vi "运维调试_五参数.vi"() -> ()   [LabVIEW 2016, in "斯坦道多参数.lvlib"]
uses:
  <vilib>/Utility/miscctls.llb/LVPointTypeDef.ctl
  <vilib>/Utility/config.llb/NI_LVConfig.lvlib
panel:
  out "运行状态":u16(ring) items=["空闲", "水样测试", "标样核查"]
  in  "叶绿素a校准":bool
  in  "停止":bool
  in  "标样核查":bool
  in  "水样测试":bool
  in  "open MB":bool
  in  "设置":bool
  in  "水温校准":bool
  in  "浊度校准":bool
  in  "溶解氧校准":bool
  in  "电导率校准":bool
  in  "pH校准":bool
  in  "探头校正返回":bool
  in  "探头校正":bool
  out "检测值":T1
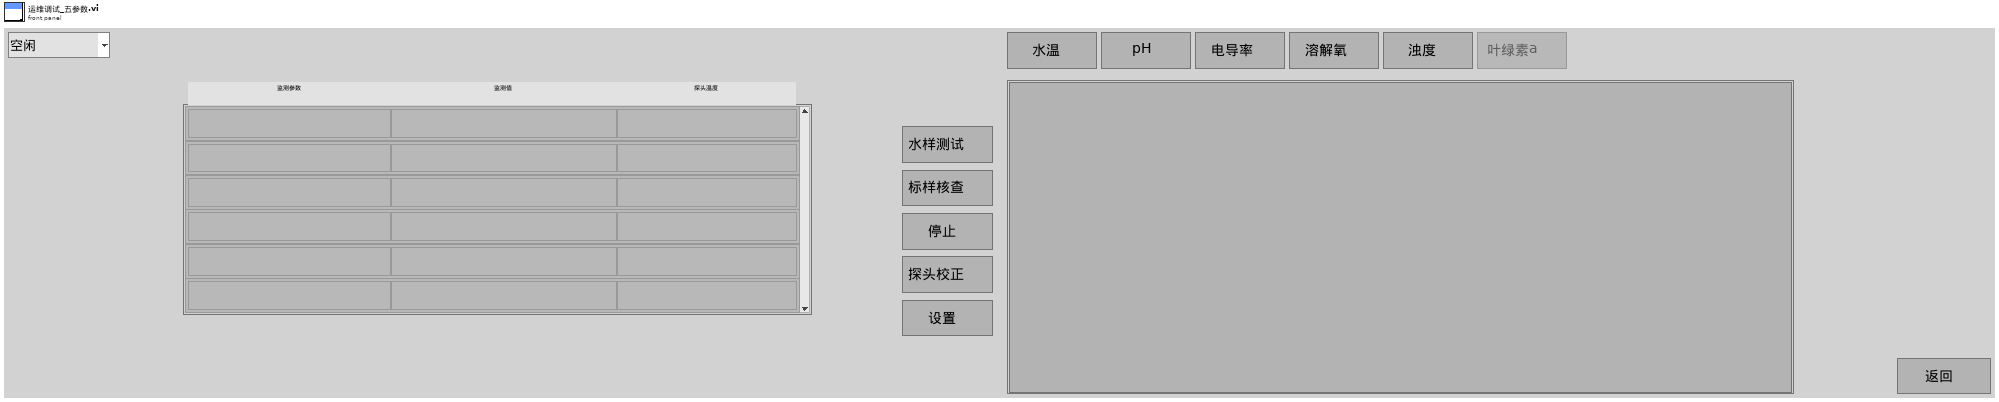
[diagram p1: front panel]
types:
  T1 = typedef "斯坦道多参数.lvlib/检测值.ctl" = cluster{"监测参数1":string, "浓度1":string, "探头温度1":string}[]
  T2 = typedef "LVPointTypeDef.ctl" = cluster{"Horizontal":i16, "Vertical":i16}
  T3 = cluster{"电极状态标志":u16, "电极型号标志":u16, "酸碱度测量值":sgl, "温度测量值":sgl, "酸碱度信号值":sgl, "温度信号值":sgl, "酸碱度偏移修正值":sgl, "温度偏移修正值":sgl, "手动温度补偿值":sgl, "酸碱度电极零点":sgl, "酸碱度电极斜率":sgl, "第1点标准值记录":sgl, "第1点信号值记录":sgl, "第1点温度值记录":sgl, "第2点标准值记录":sgl, "第2点信号值记录":sgl, "第2点温度值记录":sgl, "命令滤波设定":u16, "温度模式":enum16{"ATC", "MTC"}, "生产批次":u16, "电极序号":u16, "串口地址":u16, "串口波特率":enum16{"9600", "19200", "115200"}, "串口校验位":enum16{"NONE", "ODD", "EVEN"}, "串口停止位":enum16{"1bit", "2bit"}, "第一点标准值":sgl, "第二点标准值":sgl}
  T4 = cluster{"电极状态标志":u16, "电极型号标志":u16, "电导率测量值":sgl, "温度测量值":sgl, "电导率信号值":sgl, "温度信号值":sgl, "温度补偿系数":sgl, "电导率偏移修正值":sgl, "温度偏移修正值":sgl, "手动温度补偿值":sgl, "电导率电极零点":sgl, "电导率电极斜率":sgl, "命令滤波设定":u16, "温度模式":enum16{"ATC", "MTC"}, "生产批次":u16, "电极序号":u16, "串口地址":u16, "串口波特率":enum16{"9600", "19200", "115200"}, "串口校验位":enum16{"NONE", "ODD", "EVEN"}, "串口停止位":enum16{"1bit", "2bit"}, "第一点标准值":sgl, "第二点标准值":sgl}
  T5 = cluster{"监测参数1":string, "浓度1":string, "探头温度1":string}[]
  T6 = enum8{"Enabled", "Disabled", "Disabled and Grayed Out"}
  T7 = cluster{"CH":u16, "监测值":dbl, "监测信号值":dbl, "温度偏移修正值":sgl}
  T8 = typedef "NI_LVConfig.lvlib/Config Data RefNum.ctl" = refnum<k1>
  T9 = cluster{"baud rate (bps)":u32, "stop bits":u16, "parity":u16, "flow control":u16, "timeout":u32, "retries":i32}
  T10 = enum32{"Bad", "Idle", "Run top level", "Running"}
  T11 = cluster{"数据保存间隔":dbl, "水温标样值":dbl, "pH标样值":dbl, "溶解氧标样值":dbl, "电导率标样值":dbl, "浊度标样值":dbl}
  T12 = cluster{"Temp":bool, "pH":bool, "DO":bool, "Cond":bool, "Turb":bool, "叶绿素a启用":bool}
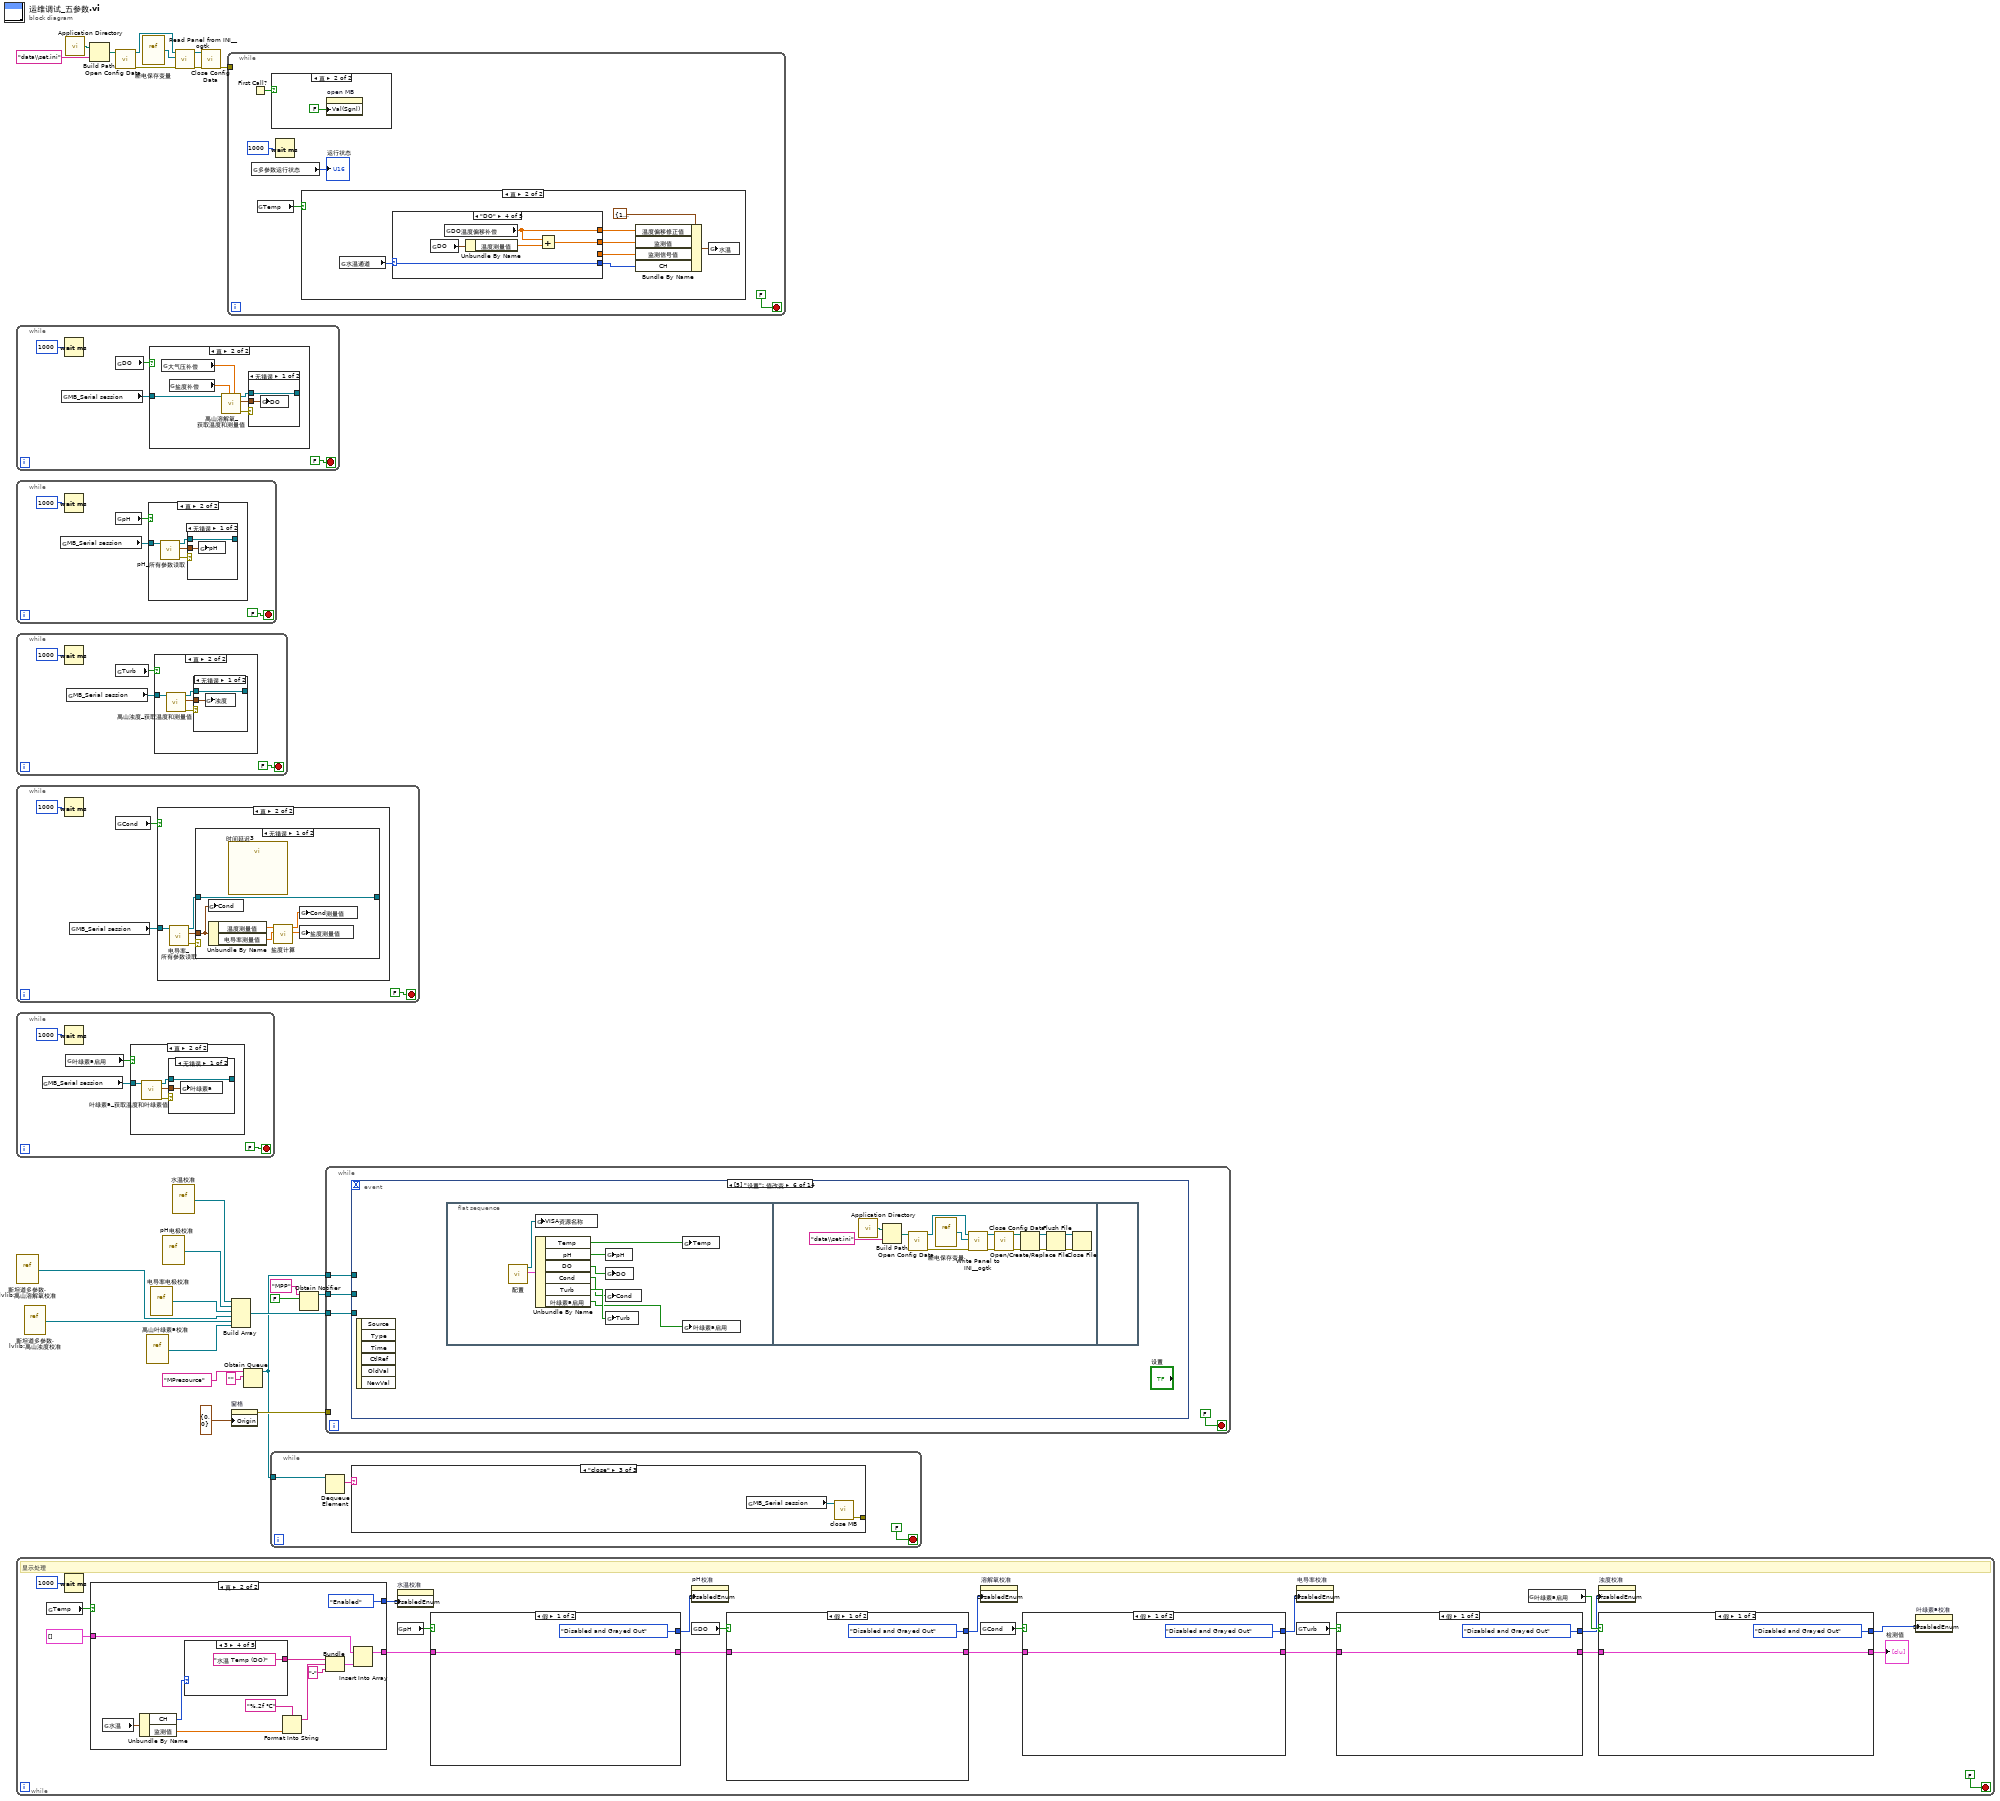
[diagram p0: block diagram]
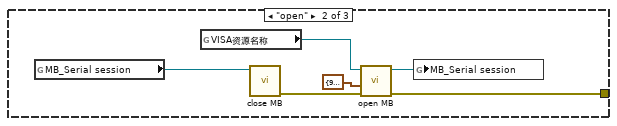
[diagram p3: hidden frame]
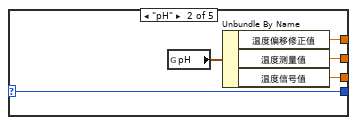
[diagram p16: hidden frame]
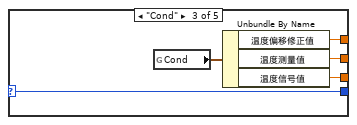
[diagram p17: hidden frame]
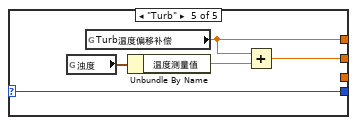
[diagram p18: hidden frame]
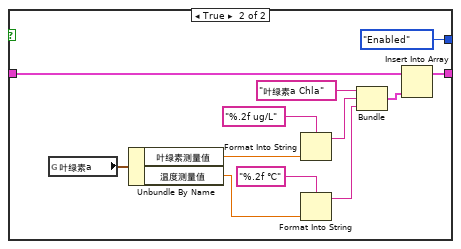
[diagram p20: hidden frame]
diagram:
  n1 = while {
    stop <- FALSE stop-if-true
    n2 = global read "多参数全局变量.vi" "MB_Serial session"() -> (w25:refnum<class "MB_Master_Serial.lvclass">)
    n3 = Wait (ms)(milliseconds to wait=u32 1000 ("等待时间（毫秒）")) -> ()  [unwired: 1 out]
    n4 = global read "断电保存变量.vi" "DO"() -> (w26:bool)
    n5 = case shown="真" w26 {
      tunnel: w25 -> [_ w31]
      frame False {
      }
      frame True {
        n6 = global read "断电保存变量.vi" "大气压补偿"() -> (w30:dbl)
        n7 = global read "断电保存变量.vi" "盐度补偿"() -> (w29:dbl)
        n8 = call "禹山溶解氧_获取温度和测量值.vi"("大气压补偿"=w30, "盐度补偿"=w29, "MB_Serial session in"=w31) -> ("error out"=w33:errorcluster, "输出值"=w34:cluster{"温度测量值":sgl, "DO%":sgl, "DOmg/L":sgl}, "MB_Serial session out"=w32:refnum<class "MB_Master_Serial.lvclass">)  [unwired: 6 in]
        n9 = case shown="无错误" w33 {
          tunnel: w34 -> [w35 _]
          tunnel: w32 -> [w36 w37]
          tunnel: [w36 w37] -> _
          frame No Error {
            n10 = global write "禹山过程全局变量.vi" "DO"(w35) -> ()
          }
          frame Error {
          }
        }
      }
    }
  }
  n11 = while {
    stop <- FALSE stop-if-true
    n12 = global read "多参数全局变量.vi" "MB_Serial session"() -> (w38:refnum<class "MB_Master_Serial.lvclass">)
    n13 = Wait (ms)(milliseconds to wait=u32 1000 ("等待时间（毫秒）")) -> ()  [unwired: 1 out]
    n14 = global read "断电保存变量.vi" "pH"() -> (w40:bool)
    n15 = case shown="真" w40 {
      tunnel: w38 -> [_ w42]
      frame False {
      }
      frame True {
        n16 = call "pH_所有参数读取.vi"("MB_Serial session in"=w42) -> ("error out"=w44:errorcluster, "输出值"=w45:T3, "MB_Serial session out"=w43:refnum<class "MB_Master_Serial.lvclass">)  [unwired: 8 in]
        n17 = case shown="无错误" w44 {
          tunnel: w45 -> [w47 _]
          tunnel: w43 -> [w46 w48]
          tunnel: [w46 w48] -> _
          frame No Error {
            n18 = global write "国弘过程全局变量.vi" "pH"(w47) -> ()
          }
          frame Error {
          }
        }
      }
    }
  }
  n19 = while {
    stop <- FALSE stop-if-true
    n20 = Wait (ms)(milliseconds to wait=u32 1000 ("等待时间（毫秒）")) -> ()  [unwired: 1 out]
    n21 = global read "多参数全局变量.vi" "MB_Serial session"() -> (w49:refnum<class "MB_Master_Serial.lvclass">)
    n22 = global read "断电保存变量.vi" "Turb"() -> (w51:bool)
    n23 = case shown="真" w51 {
      tunnel: w49 -> [_ w53]
      frame False {
      }
      frame True {
        n24 = call "禹山浊度_获取温度和测量值.vi"("MB_Serial session in"=w53) -> ("error out"=w55:errorcluster, "输出值"=w56:cluster{"温度测量值":sgl, "浊度":sgl}, "MB_Serial session out"=w54:refnum<class "MB_Master_Serial.lvclass">)  [unwired: 8 in]
        n25 = case shown="无错误" w55 {
          tunnel: w56 -> [w57 _]
          tunnel: w54 -> [w58 w59]
          tunnel: [w58 w59] -> _
          frame No Error {
            n26 = global write "禹山过程全局变量.vi" "浊度"(w57) -> ()
          }
          frame Error {
          }
        }
      }
    }
  }
  n27 = while {
    stop <- FALSE stop-if-true
    n28 = Wait (ms)(milliseconds to wait=u32 1000 ("等待时间（毫秒）")) -> ()  [unwired: 1 out]
    n29 = global read "多参数全局变量.vi" "MB_Serial session"() -> (w60:refnum<class "MB_Master_Serial.lvclass">)
    n30 = global read "断电保存变量.vi" "Cond"() -> (w62:bool)
    n31 = case shown="真" w62 {
      tunnel: w60 -> [_ w64]
      frame False {
      }
      frame True {
        n32 = call "电导率_所有参数读取.vi"("MB_Serial session in"=w64) -> ("error out"=w66:errorcluster, "输出值"=w67:T4, "MB_Serial session out"=w65:refnum<class "MB_Master_Serial.lvclass">)  [unwired: 8 in]
        n33 = case shown="无错误" w66 {
          tunnel: w67 -> [w72 _]
          tunnel: [w73 w74] -> _
          tunnel: w65 -> [w73 w74]
          frame No Error {
            n34 = global write "国弘过程全局变量.vi" "Cond"(w72) -> ()
            n35 = Unbundle By Name(w72) -> ("温度测量值"=w70:sgl, "电导率测量值"=w71:sgl)
            n36 = call "时间延迟3"() -> ()  [unwired: 11 in, 1 out]
            n37 = call "盐度计算.vi"("spCond"=w71, "Temp"=w70) -> ("saltresult"=w68:dbl, "cond"=w69:dbl)  [unwired: 8 in]
            n38 = global write "国弘过程全局变量.vi" "Cond测量值"(w69) -> ()
            n39 = global write "国弘过程全局变量.vi" "盐度测量值"(w68) -> ()
          }
          frame Error {
          }
        }
      }
    }
  }
  n40 = while {
    stop <- FALSE stop-if-true
    n41 = global read "多参数全局变量.vi" "MB_Serial session"() -> (w75:refnum<class "MB_Master_Serial.lvclass">)
    n42 = Wait (ms)(milliseconds to wait=u32 1000 ("等待时间（毫秒）")) -> ()  [unwired: 1 out]
    n43 = global read "断电保存变量.vi" "叶绿素a启用"() -> (w77:bool)
    n44 = case shown="真" w77 {
      tunnel: w75 -> [_ w79]
      frame False {
      }
      frame True {
        n45 = call "叶绿素a_获取温度和叶绿素值.vi"("MB_Serial session in"=w79) -> ("error out"=w81:errorcluster, "输出值"=w82:cluster{"温度测量值":sgl, "叶绿素测量值":sgl, "错误标志":u16}, "MB_Serial session out"=w80:refnum<class "MB_Master_Serial.lvclass">)  [unwired: 8 in]
        n46 = case shown="无错误" w81 {
          tunnel: w82 -> [w83 _]
          tunnel: w80 -> [w84 w85]
          tunnel: [w84 w85] -> _
          frame No Error {
            n47 = global write "禹山过程全局变量.vi" "叶绿素a"(w83) -> ()
          }
          frame Error {
          }
        }
      }
    }
  }
  n48 = vi-ref "斯坦道多参数.lvlib:禹山溶解氧校准.vi"() -> (w18:refnum<vi>)
  n49 = while {
    stop <- FALSE stop-if-true
    # "显示处理"
    n50 = global read "断电保存变量.vi" "Temp"() -> (w104:bool)
    n51 = Wait (ms)(milliseconds to wait=u32 1000 ("等待时间（毫秒）")) -> ()  [unwired: 1 out]
    n52 = case shown="真" w104 {
      tunnel: [w182 w184] -> w101
      tunnel: T5 [] ("数组") -> [w182 w185]
      tunnel: [T6."Disabled and Grayed Out" ("禁用") T6."Enabled" ("禁用")] -> w86
      frame False {
      }
      frame True {
        n53 = global read "国弘过程全局变量.vi" "水温"() -> (w193:T7)
        n54 = Unbundle By Name(w193) -> ("CH"=w190:u16, "监测值"=w191:dbl)
        n55 = case shown="3" w190 {
          tunnel: ["水温 Temp" ("监测参数1") "水温 Temp (pH)" ("监测参数1") "水温 Temp (Cond)" ("监测参数1") "水温 Temp (DO)" ("监测参数1") "水温 Temp (Turb)" ("监测参数1")] -> w189
          frame 0, Default {
          }
          frame 1 {
          }
          frame 2 {
          }
          frame 3 {
          }
          frame 4 {
          }
        }
        n56 = Format Into String(format string="%.2f ℃" ("格式字符串"), w191) -> (resulting string=w188:string)  [unwired: 2 in, 1 out]
        n57 = Bundle("监测参数1"=w189, w188, "探头温度1"="-") -> (w186:cluster{"监测参数1":string, string, "探头温度1":string})  [unwired: 1 in]
        n58 = Insert Into Array(array=w185, new element=w186) -> (w184:T5)  [unwired: 1 in]
      }
    }
    n59 = property on="水温校准" class="Bool"("DisabledEnum"=w86) -> ()  [unwired: 2 in, 2 out]
    n60 = global read "断电保存变量.vi" "pH"() -> (w102:bool)
    n61 = case shown="假" w102 {
      tunnel: [w168 w170] -> w99
      tunnel: w101 -> [w168 w172]
      tunnel: [T6."Disabled and Grayed Out" ("禁用") T6."Enabled" ("禁用")] -> w91
      frame False {
      }
      frame True {
        n62 = global read "国弘过程全局变量.vi" "pH"() -> (w180:T3)
        n63 = Unbundle By Name(w180) -> ("酸碱度测量值"=w179:sgl, "温度测量值"=w177:sgl)
        n64 = Format Into String(format string="%.2f" ("格式字符串"), w179) -> (resulting string=w173:string)  [unwired: 2 in, 1 out]
        n65 = Format Into String(format string="%.2f ℃" ("格式字符串"), w177) -> (resulting string=w175:string)  [unwired: 2 in, 1 out]
        n66 = Bundle("监测参数2"="酸碱度 pH", w173, w175) -> (w171:cluster{"监测参数2":string, string, string})  [unwired: 1 in]
        n67 = Insert Into Array(array=w172, new element=w171) -> (w170:T5)  [unwired: 1 in]
      }
    }
    n68 = property on="pH校准" class="Bool"("DisabledEnum"=w91) -> ()  [unwired: 2 in, 2 out]
    n69 = global read "断电保存变量.vi" "DO"() -> (w100:bool)
    n70 = case shown="假" w100 {
      tunnel: [w150 w153] -> w96
      tunnel: w99 -> [w150 w154]
      tunnel: [T6."Disabled and Grayed Out" ("禁用") T6."Enabled" ("禁用")] -> w90
      frame False {
      }
      frame True {
        n71 = global read "禹山过程全局变量.vi" "DO"() -> (w152:cluster{"温度测量值":sgl, "DO%":sgl, "DOmg/L":sgl})
        n72 = Unbundle By Name(w152) -> ("DOmg/L"=w163:sgl, "DO%"=w161:sgl, "温度测量值"=w165:sgl)
        n73 = Format Into String(format string="%.2f mg/L" ("格式字符串"), w163) -> (resulting string=w160:string)  [unwired: 2 in, 1 out]
        n74 = Format Into String(format string="(%.2f %%)" ("格式字符串"), w161) -> (resulting string=w159:string)  [unwired: 2 in, 1 out]
        n75 = Concatenate Strings(w160, w159) -> (w158:string)
        n76 = Format Into String(format string="%.2f ℃" ("格式字符串"), w165) -> (resulting string=w156:string)  [unwired: 2 in, 1 out]
        n77 = Bundle("监测参数2"="溶解氧 DO", w158, w156) -> (w155:cluster{"监测参数2":string, string, string})  [unwired: 1 in]
        n78 = Insert Into Array(array=w154, new element=w155) -> (w153:T5)  [unwired: 1 in]
      }
    }
    n79 = property on="溶解氧校准" class="Bool"("DisabledEnum"=w90) -> ()  [unwired: 2 in, 2 out]
    n80 = global read "断电保存变量.vi" "Cond"() -> (w98:bool)
    n81 = case shown="假" w98 {
      tunnel: w96 -> [w136 w140]
      tunnel: [w136 w138] -> w95
      tunnel: [T6."Disabled and Grayed Out" ("禁用") T6."Enabled" ("禁用")] -> w89
      frame False {
      }
      frame True {
        n82 = global read "国弘过程全局变量.vi" "Cond"() -> (w148:T4)
        n83 = Unbundle By Name(w148) -> ("电导率测量值"=w147:sgl, "温度测量值"=w145:sgl)
        n84 = Format Into String(format string="%.2f uS/cm" ("格式字符串"), w147) -> (resulting string=w141:string)  [unwired: 2 in, 1 out]
        n85 = Format Into String(format string="%.2f ℃" ("格式字符串"), w145) -> (resulting string=w142:string)  [unwired: 2 in, 1 out]
        n86 = Bundle("监测参数2"="电导率 Cond", w141, w142) -> (w139:cluster{"监测参数2":string, string, string})  [unwired: 1 in]
        n87 = Insert Into Array(array=w140, new element=w139) -> (w138:T5)  [unwired: 1 in]
      }
    }
    n88 = property on="电导率校准" class="Bool"("DisabledEnum"=w89) -> ()  [unwired: 2 in, 2 out]
    n89 = global read "断电保存变量.vi" "Turb"() -> (w97:bool)
    n90 = case shown="假" w97 {
      tunnel: w95 -> [w122 w127]
      tunnel: [w122 w125] -> w94
      tunnel: [T6."Disabled and Grayed Out" ("禁用") T6."Enabled" ("禁用")] -> w88
      frame False {
      }
      frame True {
        n91 = global read "禹山过程全局变量.vi" "浊度"() -> (w124:cluster{"温度测量值":sgl, "浊度测量值":sgl})
        n92 = Unbundle By Name(w124) -> ("浊度测量值"=w131:sgl, "温度测量值"=w133:sgl)
        n93 = Format Into String(format string="%.2f NTU" ("格式字符串"), w131) -> (resulting string=w129:string)  [unwired: 2 in, 1 out]
        n94 = Format Into String(format string="%.2f ℃" ("格式字符串"), w133) -> (resulting string=w130:string)  [unwired: 2 in, 1 out]
        n95 = Bundle("监测参数2"="浊度 Turb", w129, w130) -> (w126:cluster{"监测参数2":string, string, string})  [unwired: 1 in]
        n96 = Insert Into Array(array=w127, new element=w126) -> (w125:T5)  [unwired: 1 in]
      }
    }
    n97 = global read "断电保存变量.vi" "叶绿素a启用"() -> (w92:bool)
    n98 = property on="浊度校准" class="Bool"("DisabledEnum"=w88) -> ()  [unwired: 2 in, 2 out]
    n99 = case shown="假" w92 {
      tunnel: w94 -> [w108 w115]
      tunnel: [w108 w113] -> w93
      tunnel: [T6."Disabled and Grayed Out" ("禁用") T6."Enabled" ("禁用")] -> w87
      frame False {
      }
      frame True {
        n100 = global read "禹山过程全局变量.vi" "叶绿素a"() -> (w112:cluster{"温度测量值":sgl, "叶绿素测量值":sgl, "错误标志":u16})
        n101 = Unbundle By Name(w112) -> ("叶绿素测量值"=w111:sgl, "温度测量值"=w110:sgl)
        n102 = Format Into String(format string="%.2f ug/L" ("格式字符串"), w111) -> (resulting string=w117:string)  [unwired: 2 in, 1 out]
        n103 = Format Into String(format string="%.2f ℃" ("格式字符串"), w110) -> (resulting string=w118:string)  [unwired: 2 in, 1 out]
        n104 = Bundle("监测参数2"="叶绿素a Chla", w117, w118) -> (w114:cluster{"监测参数2":string, string, string})  [unwired: 1 in]
        n105 = Insert Into Array(array=w115, new element=w114) -> (w113:T5)  [unwired: 1 in]
      }
    }
    "检测值" <- w93
    n106 = property on="叶绿素a校准" class="Bool"("DisabledEnum"=w87) -> ()  [unwired: 2 in, 2 out]
  }
  n107 = vi-ref "斯坦道多参数.lvlib:禹山浊度校准.vi"() -> (w17:refnum<vi>)
  n108 = call <vilib>:"Application Directory.vi"() -> ("Application Directory"=w12:path)
  n109 = Build Path(base path=w12, name or relative path="data\\set.ini" ("名称或相对路径")) -> (appended path=w11:path)
  n110 = call <vilib>:"Open Config Data.vi"("configuration file path"=w11) -> ("error out"=w15:errorcluster, "refnum"=w16:T8)  [unwired: 8 in, 1 out]
  n111 = vi-ref "断电保存变量.vi"() -> (w9:refnum<vi>)
  n112 = vi-ref "禹山叶绿素a校准.vi"() -> (w7:refnum<vi>)
  n113 = vi-ref "电导率电极校准.vi"() -> (w19:refnum<vi>)
  n114 = vi-ref "pH电极校准.vi"() -> (w20:refnum<vi>)
  n115 = vi-ref "水温校准.vi"() -> (w21:refnum<vi>)
  n116 = call <userlib>:"Read Panel from INI__ogtk.vi"("error in (no error)"=w15, "VI ref"=w9, "refnum"=w16) -> ("error out"=w13:errorcluster, "refnum out"=w14:T8)  [unwired: 7 in]
  n117 = call <vilib>:"Close Config Data.vi"("error in (no error)"=w13, "refnum"=w14) -> ("error out"=w8:errorcluster)  [unwired: 8 in, 1 out]
  n118 = while {
    tunnel: w8 -> [_]
    stop <- FALSE stop-if-true
    n119 = First Call?() -> (First Call?: T/F=w201:bool)
    n120 = global read "多参数全局变量.vi" "多参数运行状态"() -> (→"运行状态":u16)
    n121 = global read "断电保存变量.vi" "Temp"() -> (w200:bool)
    n122 = case shown="真" w201 {
      frame False {
      }
      frame True {
        n123 = property on="open MB" class="Bool (严格)"("Val(Sgnl)"=FALSE ("值(信号)")) -> ()  [unwired: 2 in, 2 out]
      }
    }
    n124 = Wait (ms)(milliseconds to wait=u32 1000 ("等待时间（毫秒）")) -> ()  [unwired: 1 out]
    n125 = case shown="真" w200 {
      frame False {
      }
      frame True {
        n126 = global read "断电保存变量.vi" "水温通道"() -> (w210:enum16{"NULL", "pH", "Cond", "DO", "Turb"})
        n127 = case shown="\"DO\"" w210 {
          selector: w210 -> [w211 w216 w221 w226 w231]
          tunnel: [w211 w216 w221 w226 w231] -> w209
          tunnel: [_ w214 w219 w222 w227] -> w208
          tunnel: [_ w213 w218 _ _] -> w207
          tunnel: [_ w212 w217 w223 w229] -> w204
          frame "NULL", Default {
          }
          frame "pH" {
            n128 = global read "国弘过程全局变量.vi" "pH"() -> (w215:T3)
            n129 = Unbundle By Name(w215) -> ("温度偏移修正值"=w212:sgl, "温度测量值"=w214:sgl, "温度信号值"=w213:sgl)
          }
          frame "Cond" {
            n130 = global read "国弘过程全局变量.vi" "Cond"() -> (w220:T4)
            n131 = Unbundle By Name(w220) -> ("温度偏移修正值"=w217:sgl, "温度测量值"=w219:sgl, "温度信号值"=w218:sgl)
          }
          frame "DO" {
            n132 = global read "禹山过程全局变量.vi" "DO"() -> (w225:cluster{"温度测量值":sgl, "DO%":sgl, "DOmg/L":sgl})
            n133 = global read "断电保存变量.vi" "DO温度偏移补偿"() -> (w223:dbl)
            n134 = Unbundle By Name(w225) -> ("温度测量值"=w224:sgl)
            n135 = Add(x=w223, y=w224) -> (x+y=w222:dbl)
          }
          frame "Turb" {
            n136 = global read "禹山过程全局变量.vi" "浊度"() -> (w230:cluster{"温度测量值":sgl, "浊度测量值":sgl})
            n137 = global read "断电保存变量.vi" "Turb温度偏移补偿"() -> (w229:dbl)
            n138 = Unbundle By Name(w230) -> ("温度测量值"=w228:sgl)
            n139 = Add(x=w229, y=w228) -> (x+y=w227:dbl)
          }
        }
        n140 = Bundle By Name(cluster=T7 {"CH"=1, "监测值"=0.0, "监测信号值"=0.0, "温度偏移修正值"=0.0} ("水温"), "温度偏移修正值"=w204, "监测值"=w208, "监测信号值"=w207, "CH"=w209) -> (w206:T7)
        n141 = global write "国弘过程全局变量.vi" "水温"(w206) -> ()
      }
    }
  }
  n142 = Build Array(w21, w20, w19, w18, w17, w7) -> (w22:refnum<vi>[])
  n143 = property on="窗格" class="Pane"("Origin"=T2 {"Horizontal"=0, "Vertical"=0} ("原点")) -> (error out=w24:errorcluster)  [unwired: 2 in, 1 out]
  n144 = Obtain Queue(name (unnamed)="MPresource" ("名称（未命名）"), element data type="" ("名称（未命名）")) -> (queue out=w1:refnum<queue>)  [unwired: 3 in, 2 out]
  n145 = while {
    tunnel: w1 -> [w234]
    stop <- FALSE stop-if-true
    n146 = Dequeue Element(queue=w234) -> (element=w233:string)  [unwired: 2 in, 3 out]
    n147 = case shown="\"close\"" w233 {
      tunnel: [_ w238 w243] -> _
      frame "假", Default {
      }
      frame "open" {
        n148 = global read "多参数全局变量.vi" "MB_Serial session"() -> (w237:refnum<class "MB_Master_Serial.lvclass">)
        n149 = global read "断电保存变量.vi" "VISA资源名称"() -> (w240:refnum<visa-resource-name>)
        n150 = call "close MB.vi"("MB_Serial session"=w237) -> ("error out"=w241:errorcluster)  [unwired: 10 in]
        n151 = call "open MB.vi"("error in (no error)"=w241, "Serial Config"=T9 {"baud rate (bps)"=9600, "stop bits"=10, "parity"=0, "flow control"=0, "timeout"=1000, "retries"=1}, "VISA资源名称"=w240) -> ("error out"=w238:errorcluster, "MB_Serial session"=w236:refnum<class "MB_Master_Serial.lvclass">)  [unwired: 7 in]
        n152 = global write "多参数全局变量.vi" "MB_Serial session"(w236) -> ()
      }
      frame "close" {
        n153 = global read "多参数全局变量.vi" "MB_Serial session"() -> (w242:refnum<class "MB_Master_Serial.lvclass">)
        n154 = call "close MB.vi"("MB_Serial session"=w242) -> ("error out"=w243:errorcluster)  [unwired: 10 in]
      }
    }
  }
  n155 = Obtain Notifier(name (unnamed)="MPP" ("名称（未命名）"), notification data type=FALSE) -> (notifier out=w4:refnum<notifier>)  [unwired: 2 in, 2 out]
  n156 = while {
    tunnel: w24 -> [_]
    tunnel: w22 -> [w246]
    tunnel: w4 -> [w245]
    tunnel: w1 -> [w244]
    stop <- FALSE stop-if-true
    n157 = event shown="[5] \"设置\": 值改变" {
      selector: _ -> [_ _ _ _ _ _ _ _ _ _ _ _ _ _]
      dyn-events: _ -> [_ _ _ _ _ _ _ _ _ _ _ _ _ _]
      timeout: _ -> [_ _ _ _ _ _ _ _ _ _ _ _ _ _]
      tunnel: w246 -> [_ _ _ _ _ _ w305 w318 w331 w343 w355 w367 w379 w391]
      tunnel: w245 -> [_ _ _ w279 _ _ _ _ _ _ _ _ _ _]
      tunnel: w244 -> [_ _ _ _ w282 _ _ _ _ _ _ _ _ _]
      event Timeout {
        n158 = event-data() -> ()  [unwired: 1 in, 3 out]
      }
      event "水样测试": Value Change {
        n159 = event-data() -> ()  [unwired: 1 in, 6 out]
        n160 = call "水样测试配置.vi"() -> ("确认输出"=w249:bool, "水样测定时间输出"=w248:dbl)  [unwired: 10 in]
        n161 = case shown="真" w249 {
          tunnel: w248 -> [_ w252]
          frame False {
          }
          frame True {
            n162 = vi-ref "水样测试.vi"() -> (w253:refnum<vi>)
            n163 = property class="VI"(reference=w253) -> ("Name"=w257:string, "Exec.State"=w255:T10)  [unwired: 1 in, 2 out]
            n164 = Open VI Reference(type specifier VI Refnum (for type only)=refnum<vi> refnum, vi path=w257, options=128 ("选项")) -> (vi reference=w258:refnum<vi>)  [unwired: 3 in, 1 out]
            n165 = case shown="\"Idle\"" w255 {
              tunnel: [w259 w263] -> w254
              tunnel: w258 -> [w259 w262]
              tunnel: w252 -> [_ w261]
              tunnel: "hd" ("数据标记表") -> [_ w260]
              frame "Bad", Default {
              }
              frame "Idle" {
                n166 = call-by-ref "开始异步调用"(reference=w262, "数据标记表"=w260, "水样测试时间"=w261) -> (reference out=w263:refnum<vi>)  [unwired: 11 in, 1 out]
              }
            }
            n167 = Close Reference(reference=w254) -> ()  [unwired: 1 in, 1 out]
          }
        }
      }
      event "标样核查": Value Change {
        n168 = event-data() -> ()  [unwired: 1 in, 6 out]
        n169 = call "标样核查配置.vi"() -> ("确认输出"=w265:bool, "标样核查配置"=w264:T11)  [unwired: 10 in]
        n170 = case shown="真" w265 {
          tunnel: w264 -> [_ w266]
          frame False {
          }
          frame True {
            n171 = vi-ref "标样核查.vi"() -> (w267:refnum<vi>)
            n172 = property class="VI"(reference=w267) -> ("Name"=w272:string, "Exec.State"=w269:T10)  [unwired: 1 in, 2 out]
            n173 = Open VI Reference(type specifier VI Refnum (for type only)=refnum<vi> refnum, vi path=w272, options=128 ("选项")) -> (vi reference=w273:refnum<vi>)  [unwired: 3 in, 1 out]
            n174 = case shown="\"Idle\"" w269 {
              tunnel: [w274 w277] -> w268
              tunnel: w273 -> [w274 w276]
              tunnel: w266 -> [_ w275]
              frame "Bad", Default {
              }
              frame "Idle" {
                n175 = call-by-ref "开始异步调用"(reference=w276, "标样核查配置"=w275) -> (reference out=w277:refnum<vi>)  [unwired: 12 in, 1 out]
              }
            }
            n176 = Close Reference(reference=w268) -> ()  [unwired: 1 in, 1 out]
          }
        }
      }
      event "停止": Value Change {
        n177 = event-data() -> ()  [unwired: 1 in, 6 out]
        n178 = Send Notification(notification=TRUE ("通知"), notifier=w279) -> ()  [unwired: 1 in, 2 out]
      }
      event "open MB": Value Change {
        n179 = event-data() -> ()  [unwired: 1 in, 6 out]
        n180 = Flush Queue(queue=w282) -> (queue out=w281:refnum<queue>)  [unwired: 1 in, 2 out]
        n181 = Enqueue Element(queue=w281, element="open" ("元素")) -> ()  [unwired: 2 in, 3 out]
      }
      event "设置": Value Change {
        n182 = event-data() -> ()  [unwired: 1 in, 6 out]
        n183 = flat-sequence {
          frame #0 {
            n184 = call "配置.vi"() -> ("启用参数"=w289:T12, "串口输出"=w290:refnum<visa-resource-name>)  [unwired: 10 in]
            n185 = global write "断电保存变量.vi" "VISA资源名称"(w290) -> ()
            n186 = Unbundle By Name(w289) -> ("Temp"=w284:bool, "pH"=w285:bool, "DO"=w286:bool, "Cond"=w287:bool, "Turb"=w288:bool, "叶绿素a启用"=w283:bool)
            n187 = global write "断电保存变量.vi" "pH"(w285) -> ()
            n188 = global write "断电保存变量.vi" "DO"(w286) -> ()
            n189 = global write "断电保存变量.vi" "Cond"(w287) -> ()
            n190 = global write "断电保存变量.vi" "Turb"(w288) -> ()
            n191 = global write "断电保存变量.vi" "Temp"(w284) -> ()
            n192 = global write "断电保存变量.vi" "叶绿素a启用"(w283) -> ()
          }
          frame #1 {
            n193 = call <vilib>:"Application Directory.vi"() -> ("Application Directory"=w300:path)
            n194 = Build Path(base path=w300, name or relative path="data\\set.ini" ("名称或相对路径")) -> (appended path=w299:path)
            n195 = call <vilib>:"Open Config Data.vi"("configuration file path"=w299) -> ("error out"=w303:errorcluster, "refnum"=w304:T8)  [unwired: 8 in, 1 out]
            n196 = vi-ref "断电保存变量.vi"() -> (w297:refnum<vi>)
            n197 = call <userlib>:"Write Panel to INI__ogtk.vi"("error in (no error)"=w303, "VI ref"=w297, "refnum"=w304) -> ("error out"=w301:errorcluster, "refnum out"=w302:T8)  [unwired: 7 in]
            n198 = call <vilib>:"Close Config Data.vi"("error in (no error)"=w301, "refnum"=w302) -> ("error out"=w293:errorcluster, "file path"=w294:path)  [unwired: 8 in]
            n199 = Open/Create/Replace File(file path (use dialog)=w294, error in=w293) -> (refnum out=w295:refnum<file>, error out=w296:errorcluster)  [unwired: 4 in, 1 out]
            n200 = Flush File(refnum=w295, error in=w296) -> (refnum out=w291:refnum<file>, error out=w292:errorcluster)
            n201 = Close File(refnum=w291, error in=w292) -> ()  [unwired: 2 out]
          }
          frame #2 {
          }
        }
      }
      event "探头校正返回": Value Change {
        n202 = event-data() -> ()  [unwired: 1 in, 6 out]
        n203 = disable-structure shown="禁用" {
          disable-tunnel: w305 -> [w307 _]
          frame Disabled {
            n204 = for {
              tunnel: w307 -> [w310] mode=indexing
              n205 = property class="VI"(reference=w310) -> (reference out=w308:refnum<vi>, "Exec.State"=w309:T10)  [unwired: 1 in, 1 out]
              n206 = case shown="\"Run top level\"" w309 {
                tunnel: w308 -> [_ _ w311 w312]
                frame "Bad", Default {
                }
                frame "Idle" {
                }
                frame "Run top level" {
                  n207 = invoke class="VI" method="Abort VI"(reference=w311) -> ()  [unwired: 2 in, 3 out]
                }
                frame "Running" {
                  n208 = invoke class="VI" method="Abort VI"(reference=w312) -> ()  [unwired: 2 in, 3 out]
                }
              }
            }
          }
          frame Enabled {
          }
        }
        n209 = property on="窗格" class="Pane"("Origin"=T2 {"Horizontal"=0, "Vertical"=0} ("原点")) -> ()  [unwired: 2 in, 2 out]
      }
      event "探头校正": Value Change {
        n210 = event-data() -> ()  [unwired: 1 in, 6 out]
        n211 = property on="窗格" class="Pane"("Origin"=T2 {"Horizontal"=1656, "Vertical"=0} ("原点")) -> ()  [unwired: 2 in, 2 out]
        n212 = Index Array(array=w318, index=0 ("索引")) -> (element=w319:refnum<vi>)
        n213 = property class="VI"(reference=w319) -> (reference out=w314:refnum<vi>, "Exec.State"=w313:T10)  [unwired: 1 in, 1 out]
        n214 = case shown="\"Bad\", 默认" w313 {
          tunnel: [w321 w323] -> w317
          tunnel: w314 -> [w321 w322]
          frame "Bad", Default {
          }
          frame "Idle" {
            n215 = invoke class="VI" method="Run VI"(reference=w322, "Wait until done"=FALSE ("结束前等待"), "Auto Dispose Ref"=FALSE ("自动销毁引用")) -> (reference out=w323:refnum<vi>)  [unwired: 2 in, 4 out]
          }
        }
        n216 = invoke on="探头校准子面板" class="SubPnl" method="Remove VI"() -> (error out=w316:errorcluster)  [unwired: 3 in, 2 out]
        n217 = invoke on="探头校准子面板" class="SubPnl" method="Insert VI"(error in=w316, "VI Ref"=w317) -> ()  [unwired: 2 in, 4 out]
      }
      event "水温校准": Value Change {
        n218 = event-data() -> ()  [unwired: 1 in, 6 out]
        n219 = Index Array(array=w331, index=0 ("索引")) -> (element=w332:refnum<vi>)
        n220 = property class="VI"(reference=w332) -> (reference out=w327:refnum<vi>, "Exec.State"=w326:T10)  [unwired: 1 in, 1 out]
        n221 = case shown="\"Bad\", 默认" w326 {
          tunnel: [w333 w335] -> w329
          tunnel: w327 -> [w333 w334]
          frame "Bad", Default {
          }
          frame "Idle" {
            n222 = invoke class="VI" method="Run VI"(reference=w334, "Wait until done"=FALSE ("结束前等待"), "Auto Dispose Ref"=FALSE ("自动销毁引用")) -> (reference out=w335:refnum<vi>)  [unwired: 2 in, 4 out]
          }
        }
        n223 = invoke on="探头校准子面板" class="SubPnl" method="Remove VI"() -> (error out=w328:errorcluster)  [unwired: 3 in, 2 out]
        n224 = invoke on="探头校准子面板" class="SubPnl" method="Insert VI"(error in=w328, "VI Ref"=w329) -> ()  [unwired: 2 in, 4 out]
      }
      event "pH校准": Value Change {
        n225 = event-data() -> ()  [unwired: 1 in, 6 out]
        n226 = Index Array(array=w343, index=1 ("索引")) -> (element=w344:refnum<vi>)
        n227 = property class="VI"(reference=w344) -> (reference out=w339:refnum<vi>, "Exec.State"=w338:T10)  [unwired: 1 in, 1 out]
        n228 = case shown="\"Bad\", 默认" w338 {
          tunnel: w339 -> [w345 w349]
          tunnel: [w345 w346] -> w341
          frame "Bad", Default {
          }
          frame "Idle" {
            n229 = invoke class="VI" method="Run VI"(reference=w349, "Wait until done"=FALSE ("结束前等待"), "Auto Dispose Ref"=FALSE ("自动销毁引用")) -> (reference out=w346:refnum<vi>)  [unwired: 2 in, 4 out]
          }
        }
        n230 = invoke on="探头校准子面板" class="SubPnl" method="Remove VI"() -> (error out=w340:errorcluster)  [unwired: 3 in, 2 out]
        n231 = invoke on="探头校准子面板" class="SubPnl" method="Insert VI"(error in=w340, "VI Ref"=w341) -> ()  [unwired: 2 in, 4 out]
      }
      event "电导率校准": Value Change {
        n232 = event-data() -> ()  [unwired: 1 in, 6 out]
        n233 = Index Array(array=w355, index=2 ("索引")) -> (element=w356:refnum<vi>)
        n234 = property class="VI"(reference=w356) -> (reference out=w351:refnum<vi>, "Exec.State"=w350:T10)  [unwired: 1 in, 1 out]
        n235 = case shown="\"Bad\", 默认" w350 {
          tunnel: [w357 w359] -> w353
          tunnel: w351 -> [w357 w358]
          frame "Bad", Default {
          }
          frame "Idle" {
            n236 = invoke class="VI" method="Run VI"(reference=w358, "Wait until done"=FALSE ("结束前等待"), "Auto Dispose Ref"=FALSE ("自动销毁引用")) -> (reference out=w359:refnum<vi>)  [unwired: 2 in, 4 out]
          }
        }
        n237 = invoke on="探头校准子面板" class="SubPnl" method="Remove VI"() -> (error out=w352:errorcluster)  [unwired: 3 in, 2 out]
        n238 = invoke on="探头校准子面板" class="SubPnl" method="Insert VI"(error in=w352, "VI Ref"=w353) -> ()  [unwired: 2 in, 4 out]
      }
      event "溶解氧校准": Value Change {
        n239 = event-data() -> ()  [unwired: 1 in, 6 out]
        n240 = Index Array(array=w367, index=3 ("索引")) -> (element=w368:refnum<vi>)
        n241 = property class="VI"(reference=w368) -> (reference out=w363:refnum<vi>, "Exec.State"=w362:T10)  [unwired: 1 in, 1 out]
        n242 = case shown="\"Bad\", 默认" w362 {
          tunnel: [w369 w371] -> w365
          tunnel: w363 -> [w369 w370]
          frame "Bad", Default {
          }
          frame "Idle" {
            n243 = invoke class="VI" method="Run VI"(reference=w370, "Wait until done"=FALSE ("结束前等待"), "Auto Dispose Ref"=FALSE ("自动销毁引用")) -> (reference out=w371:refnum<vi>)  [unwired: 2 in, 4 out]
          }
        }
        n244 = invoke on="探头校准子面板" class="SubPnl" method="Remove VI"() -> (error out=w364:errorcluster)  [unwired: 3 in, 2 out]
        n245 = invoke on="探头校准子面板" class="SubPnl" method="Insert VI"(error in=w364, "VI Ref"=w365) -> ()  [unwired: 2 in, 4 out]
      }
      event "浊度校准": Value Change {
        n246 = event-data() -> ()  [unwired: 1 in, 6 out]
        n247 = Index Array(array=w379, index=4 ("索引")) -> (element=w380:refnum<vi>)
        n248 = property class="VI"(reference=w380) -> (reference out=w375:refnum<vi>, "Exec.State"=w374:T10)  [unwired: 1 in, 1 out]
        n249 = case shown="\"Bad\", 默认" w374 {
          tunnel: [w381 w383] -> w377
          tunnel: w375 -> [w381 w382]
          frame "Bad", Default {
          }
          frame "Idle" {
            n250 = invoke class="VI" method="Run VI"(reference=w382, "Wait until done"=FALSE ("结束前等待"), "Auto Dispose Ref"=FALSE ("自动销毁引用")) -> (reference out=w383:refnum<vi>)  [unwired: 2 in, 4 out]
          }
        }
        n251 = invoke on="探头校准子面板" class="SubPnl" method="Remove VI"() -> (error out=w376:errorcluster)  [unwired: 3 in, 2 out]
        n252 = invoke on="探头校准子面板" class="SubPnl" method="Insert VI"(error in=w376, "VI Ref"=w377) -> ()  [unwired: 2 in, 4 out]
      }
      event "叶绿素a校准": Value Change {
        n253 = event-data() -> ()  [unwired: 1 in, 6 out]
        n254 = Index Array(array=w391, index=5 ("索引")) -> (element=w392:refnum<vi>)
        n255 = property class="VI"(reference=w392) -> (reference out=w387:refnum<vi>, "Exec.State"=w386:T10)  [unwired: 1 in, 1 out]
        n256 = case shown="\"Bad\", 默认" w386 {
          tunnel: [w393 w395] -> w389
          tunnel: w387 -> [w393 w394]
          frame "Bad", Default {
          }
          frame "Idle" {
            n257 = invoke class="VI" method="Run VI"(reference=w394, "Wait until done"=FALSE ("结束前等待"), "Auto Dispose Ref"=FALSE ("自动销毁引用")) -> (reference out=w395:refnum<vi>)  [unwired: 2 in, 4 out]
          }
        }
        n258 = invoke on="探头校准子面板" class="SubPnl" method="Remove VI"() -> (error out=w388:errorcluster)  [unwired: 3 in, 2 out]
        n259 = invoke on="探头校准子面板" class="SubPnl" method="Insert VI"(error in=w388, "VI Ref"=w389) -> ()  [unwired: 2 in, 4 out]
      }
    }
  }
